vi "MainControl.vi"(9 "Slide":refnum<vi>, 10 "notifier in":refnum<notifier>, 11 "queue in":refnum<queue>) -> ()   [LabVIEW 2013, in "main.lvlib"]
uses:
  main.lvlib
  Controls/Enum User Events.ctl
  <vilib>/DAQmx/write.llb/DAQmx Write (Digital 1D Bool NChan 1Samp 1Line).vi
  <vilib>/DAQmx/create/channels.llb/DAQmx Create Channel (DO-Digital Output).vi
  <vilib>/DAQmx/miscellaneous.llb/DAQmx Fill In Error Info.vi
  Globals/DataAcqRecordPathGlobal.vi
panel:
  in  "Offset":dbl
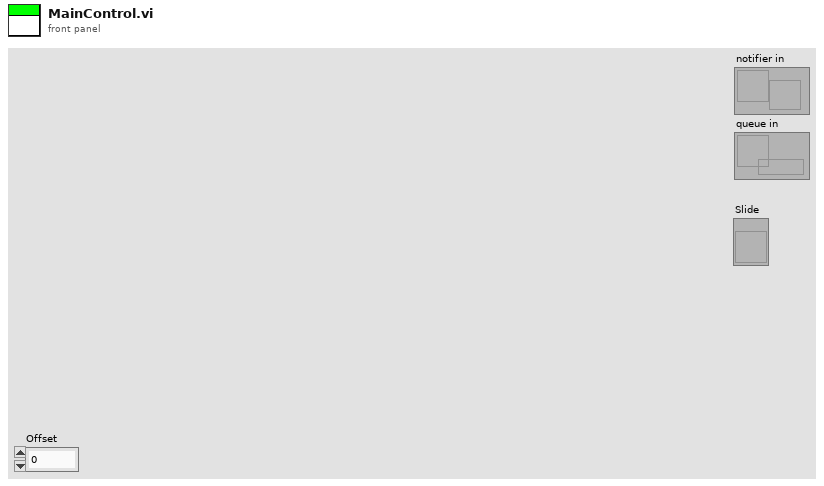
[diagram p1: front panel]
types:
  T1 = typedef "main.lvlib/Enum User Events.ctl" = enum16{"User Event", "Init"}
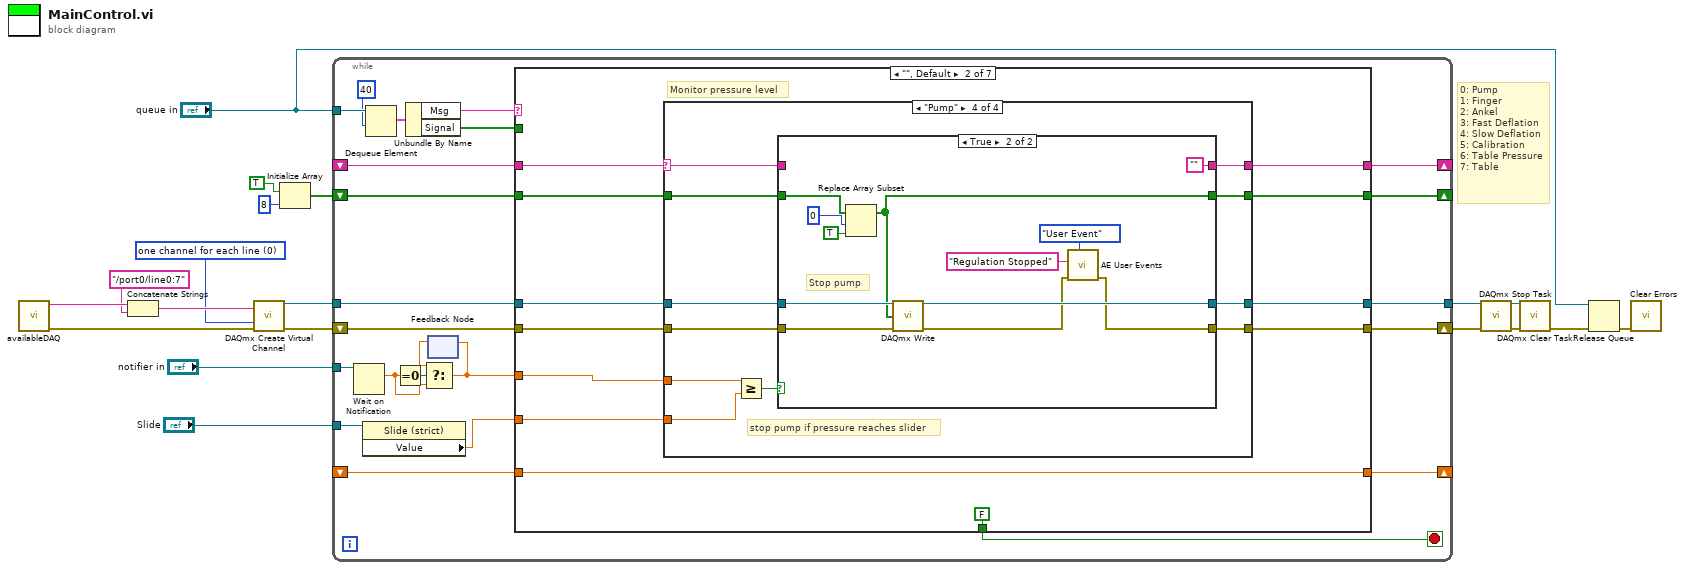
[diagram p0: block diagram]
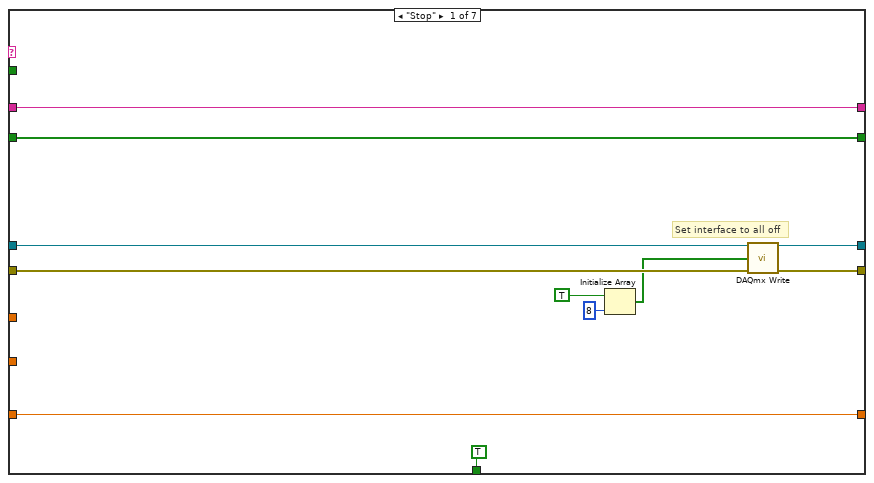
[diagram p2: hidden frame]
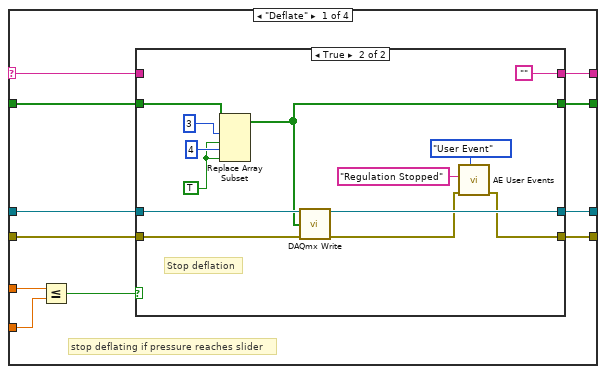
[diagram p3: hidden frame]
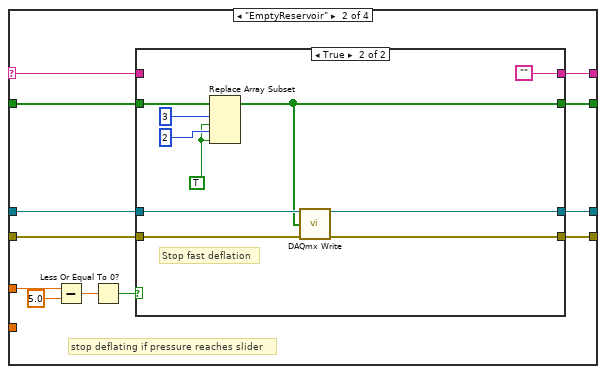
[diagram p5: hidden frame]
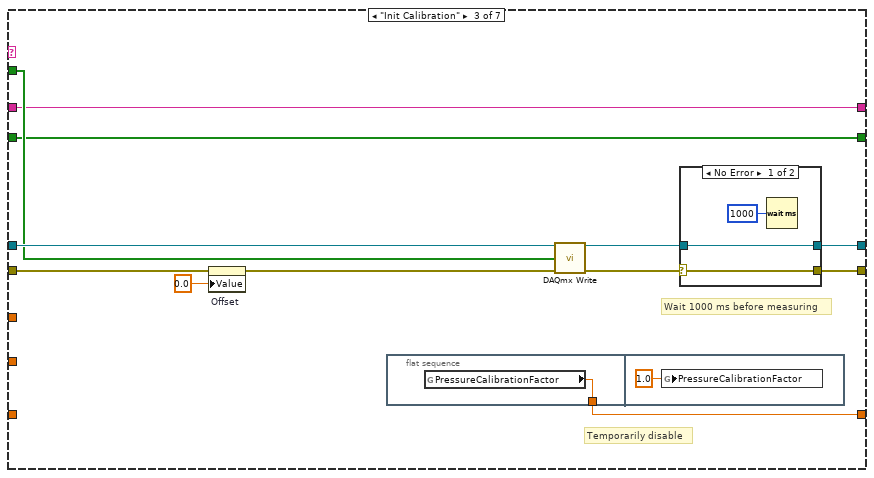
[diagram p9: hidden frame]
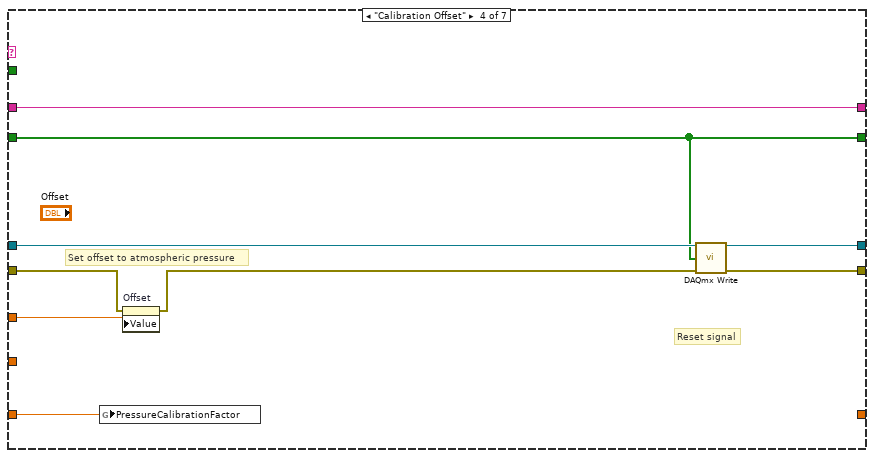
[diagram p11: hidden frame]
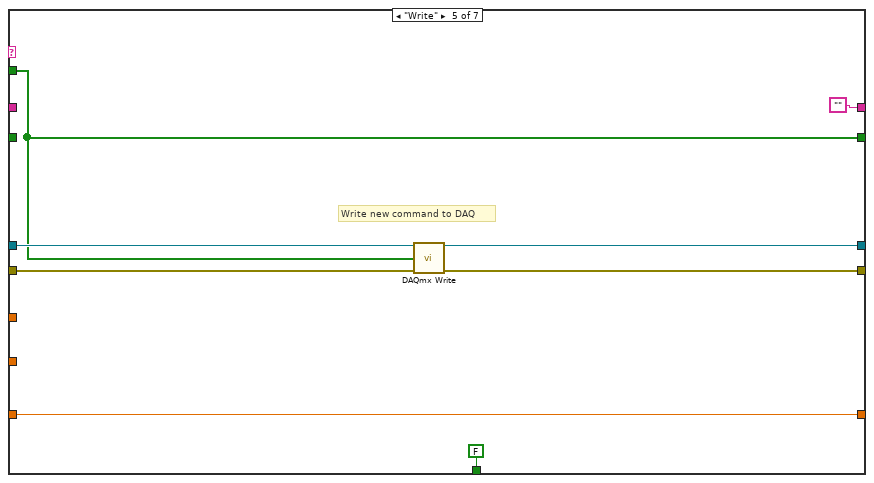
[diagram p12: hidden frame]
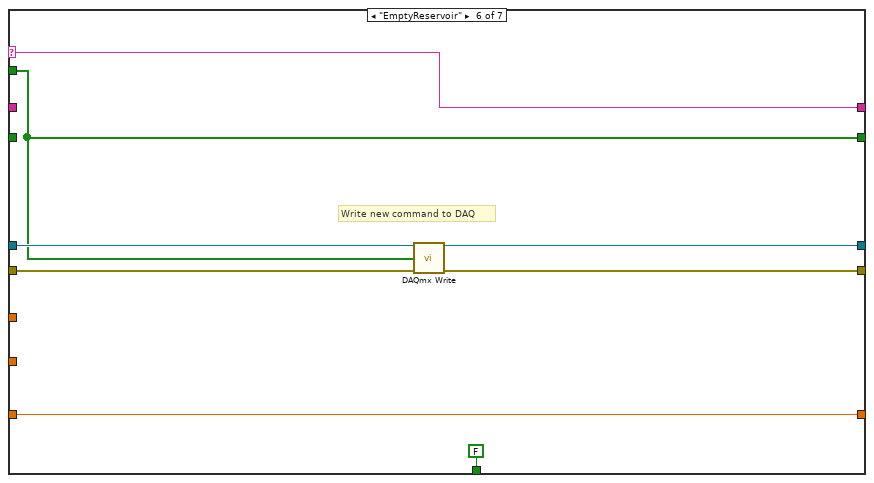
[diagram p13: hidden frame]
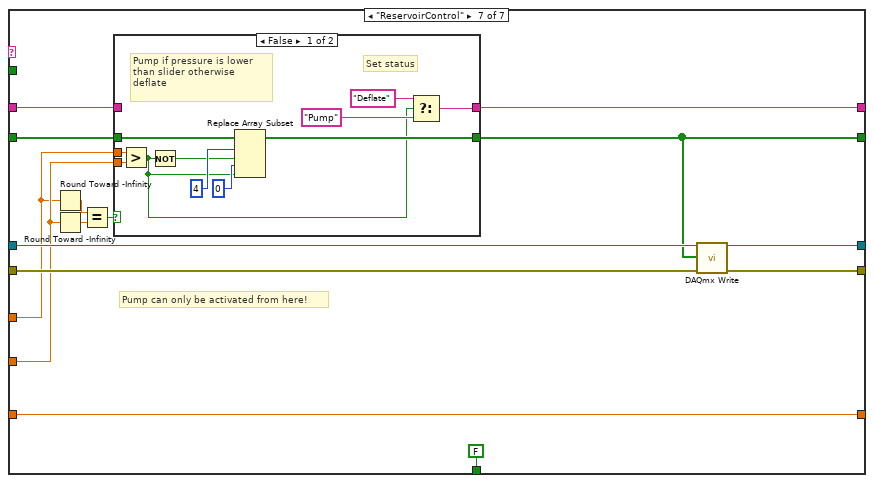
[diagram p14: hidden frame]
diagram:
  w9 = 0 items=["one channel for each line", "one channel for all lines"] ("line grouping")
  # "0: Pump\n1: Finger\n2: Ankel\n3: Fast Deflation\n4: Slow Deflation\n5: Calibration\n6: Table Pressure\n7: Table"
  n1 = call "availableDAQ.vi"() -> ("error out"=w17:errorcluster, "DAQmx Device Name"=w19:tag)  [unwired: 10 in]
  n2 = Concatenate Strings(w19, "/port0/line0:7" ("string")) -> (w16:string)
  n3 = call-poly <vilib>:"DAQmx Create Virtual Channel.vi"("lines"=w16, "line grouping"=w9, "error in"=w17) -> ("task out"=w15:refnum<k21>, "error out"=w14:errorcluster)  [unwired: 11 in]
  n4 = Initialize Array(TRUE, 8 ("dimension size")) -> (w4:bool[])
  n5 = while {
    tunnel: "queue in" -> [w42]
    tunnel: w15 -> [w41]
    shift-right: [w39] -> w12
    shift-left: w14 -> [w40]
    tunnel: [w38] -> w13
    shift-right: [w33] -> _
    shift-left: w4 -> [w32]
    shift-right: [w30] -> _
    shift-left: _ -> [w31]
    shift-right: [w29] -> _
    shift-left: _ -> [w28]
    tunnel: "notifier in" -> [w26]
    tunnel: "Slide" -> [w21]
    stop <- w35 stop-if-true
    n6 = Wait on Notification(notifier=w26) -> (notification=w24:dbl)  [unwired: 3 in, 3 out]
    n7 = property class="Slide (strict)"(reference=w21) -> ("Value"=w20:ext)  [unwired: 1 in, 2 out]
    n8 = Dequeue Element(queue=w42, timeout in ms (-1)=40) -> (element=w37:cluster{"Msg":string, "Signal":bool[]})  [unwired: 1 in, 3 out]
    n9 = Equal To 0?(x=w24) -> (x = 0?=w25:bool)
    n10 = Unbundle By Name(w37) -> ("Msg"=w36:string, "Signal"=w27:bool[])
    n11 = feedback #1() -> (w22:dbl)  [unwired: 1 in]
    n12 = Select(t=w22, s=w25, f=w24) -> (s? t:f=w23:dbl)
    n13 = feedback-in #1(w23) -> ()
    n14 = case shown="\"\", Default" w36 {
      selector: w36 -> [_ _ _ _ _ w188 _]
      tunnel: w41 -> [w49 w64 w162 w175 w186 w194 w209]
      tunnel: w40 -> [w48 w63 w154 w172 w185 w193 w208]
      tunnel: [w50 w61 w157 w176 w183 w191 w206] -> w39
      tunnel: [w51 w62 w155 w177 w184 w192 w207] -> w38
      tunnel: [TRUE FALSE _ _ FALSE FALSE FALSE] -> w35
      tunnel: w27 -> [_ _ w161 _ w181 w189 _]
      tunnel: [w52 w59 w159 w174 w181 w189 w198] -> w33
      tunnel: w32 -> [w52 w60 w159 w174 _ _ w199]
      tunnel: w31 -> [w44 w58 w160 w178 _ _ w196]
      tunnel: w23 -> [_ w57 _ w173 _ _ w200]
      tunnel: w20 -> [_ w56 _ _ _ _ w202]
      tunnel: [w44 w55 w160 w178 "" w188 w197] -> w30
      tunnel: [w43 w54 w151 _ w179 w187 w195] -> w29
      tunnel: w28 -> [w43 w54 _ w170 w179 w187 w195]
      frame "Stop" {
        # "Set interface to all off"
        n15 = Initialize Array(TRUE, 8 ("dimension size")) -> (w45:bool[])
        n16 = call-poly <vilib>:"DAQmx Write.vi"("task/channels in"=w49, "data"=w45, "error in"=w48) -> ("task out"=w51:refnum<k21>, "error out"=w50:errorcluster)  [unwired: 10 in, 1 out]
      }
      frame "", Default {
        # "Monitor pressure level"
        n17 = case shown="\"Pump\"" w58 {
          selector: w58 -> [w67 w98 w123 w125]
          tunnel: w64 -> [w71 w100 w121 w134]
          tunnel: w63 -> [w72 w101 w120 w133]
          tunnel: [w74 w103 w121 w132] -> w62
          tunnel: [w73 w102 w120 w131] -> w61
          tunnel: w60 -> [w76 w105 w122 w129]
          tunnel: [w75 w104 w122 w128] -> w59
          tunnel: [w68 w99 w123 w124] -> w55
          tunnel: w57 -> [w69 w96 _ w127]
          tunnel: w56 -> [w70 _ _ w126]
          frame "Deflate" {
            # "stop deflating if pressure reaches slider"
            n18 = Less Or Equal?(x=w69, y=w70) -> (x <= y?=w66:bool)
            n19 = case shown="True" w66 {
              tunnel: w71 -> [w80 w93]
              tunnel: w72 -> [w79 w92]
              tunnel: [w80 w91] -> w74
              tunnel: [w79 w84] -> w73
              tunnel: w76 -> [w78 w90]
              tunnel: [w78 w81] -> w75
              tunnel: [w77 ""] -> w68
              tunnel: w67 -> [w77 _]
              frame False {
              }
              frame True {
                w82 = TRUE ("new element/subarray")
                # "Stop deflation"
                n20 = Replace Array Subset(array=w90, new element #1=w82, index #1=3 ("index"), new element #2=w82, index #2=4) -> (w81:bool[])
                n21 = call-poly <vilib>:"DAQmx Write.vi"("task/channels in"=w93, "data"=w81, "error in"=w92) -> ("task out"=w91:refnum<k21>, "error out"=w85:errorcluster)  [unwired: 10 in, 1 out]
                n22 = call "AE User Events.vi"("Action"=Enum_User_Events."User Event", "error in (no error)"=w85, "User Event"="Regulation Stopped") -> ("error out"=w84:errorcluster)  [unwired: 7 in, 1 out]
              }
            }
          }
          frame "EmptyReservoir" {
            # "stop deflating if pressure reaches slider"
            n23 = Subtract(x=w96, y=5.0) -> (x-y=w95:dbl)
            n24 = Less Or Equal To 0?(x=w95) -> (x <= 0?=w97:bool)
            n25 = case shown="True" w97 {
              tunnel: w100 -> [w109 w119]
              tunnel: w101 -> [w108 w118]
              tunnel: [w109 w117] -> w103
              tunnel: [w108 w113] -> w102
              tunnel: w105 -> [w107 w116]
              tunnel: [w107 w110] -> w104
              tunnel: [w106 ""] -> w99
              tunnel: w98 -> [w106 _]
              frame False {
              }
              frame True {
                w111 = TRUE ("new element/subarray")
                # "Stop fast deflation"
                n26 = Replace Array Subset(array=w116, new element #1=w111, index #1=3 ("index"), new element #2=w111, index #2=2 ("index")) -> (w110:bool[])
                n27 = call-poly <vilib>:"DAQmx Write.vi"("task/channels in"=w119, "data"=w110, "error in"=w118) -> ("task out"=w117:refnum<k21>, "error out"=w113:errorcluster)  [unwired: 10 in, 1 out]
              }
            }
          }
          frame "", Default {
          }
          frame "Pump" {
            # "stop pump if pressure reaches slider"
            n28 = Greater Or Equal?(x=w127, y=w126) -> (x >= y?=w130:bool)
            n29 = case shown="True" w130 {
              tunnel: w134 -> [w138 w150]
              tunnel: w133 -> [w137 w149]
              tunnel: [w138 w148] -> w132
              tunnel: [w137 w142] -> w131
              tunnel: w129 -> [w136 w145]
              tunnel: [w136 w139] -> w128
              tunnel: w125 -> [w135 _]
              tunnel: [w135 ""] -> w124
              frame False {
              }
              frame True {
                # "Stop pump"
                n30 = Replace Array Subset(array=w145, new element=TRUE ("new element/subarray"), index=0) -> (w139:bool[])
                n31 = call-poly <vilib>:"DAQmx Write.vi"("task/channels in"=w150, "data"=w139, "error in"=w149) -> ("task out"=w148:refnum<k21>, "error out"=w143:errorcluster)  [unwired: 10 in, 1 out]
                n32 = call "AE User Events.vi"("Action"=Enum_User_Events."User Event", "error in (no error)"=w143, "User Event"="Regulation Stopped") -> ("error out"=w142:errorcluster)  [unwired: 7 in, 1 out]
              }
            }
          }
        }
      }
      frame "Init Calibration" {
        # "Temporarily disable"
        # "Wait 1000 ms before measuring"
        n33 = property on="Offset" class="DigNum (strict)"(error in=w154, "Value"=0.0 ("Offset")) -> (error out=w153:errorcluster)  [unwired: 1 in, 1 out]
        n34 = flat-sequence {
          tunnel: [w163] -> w151
          frame #0 {
            n35 = global read "DataAcqRecordPathGlobal.vi" "PressureCalibrationFactor"() -> (w163:dbl)
          }
          frame #1 {
            n36 = global write "DataAcqRecordPathGlobal.vi" "PressureCalibrationFactor"(1.0 ("PressureCalibrationFactor")) -> ()
          }
        }
        n37 = call-poly <vilib>:"DAQmx Write.vi"("task/channels in"=w162, "data"=w161, "error in"=w153) -> ("task out"=w156:refnum<k21>, "error out"=w158:errorcluster)  [unwired: 10 in, 1 out]
        n38 = case shown="No Error" w158 {
          selector: w158 -> [w167 w169]
          tunnel: [w167 w169] -> w157
          tunnel: [w166 w168] -> w155
          tunnel: w156 -> [w166 w168]
          frame No Error {
            n39 = Wait (ms)(milliseconds to wait=u32 1000) -> ()  [unwired: 1 out]
          }
          frame Error {
          }
        }
      }
      frame "Calibration Offset" {
        # "Reset signal"
        # "Set offset to atmospheric pressure"
        n40 = global write "DataAcqRecordPathGlobal.vi" "PressureCalibrationFactor"(w170) -> ()
        n41 = property on="Offset" class="DigNum (strict)"(error in=w172, "Value"=w173) -> (error out=w171:errorcluster)  [unwired: 1 in, 1 out]
        n42 = call-poly <vilib>:"DAQmx Write.vi"("task/channels in"=w175, "data"=w174, "error in"=w171) -> ("task out"=w177:refnum<k21>, "error out"=w176:errorcluster)  [unwired: 10 in, 1 out]
      }
      frame "Write" {
        # "Write new command to DAQ"
        n43 = call-poly <vilib>:"DAQmx Write.vi"("task/channels in"=w186, "data"=w181, "error in"=w185) -> ("task out"=w184:refnum<k21>, "error out"=w183:errorcluster)  [unwired: 10 in, 1 out]
      }
      frame "EmptyReservoir" {
        # "Write new command to DAQ"
        n44 = call-poly <vilib>:"DAQmx Write.vi"("task/channels in"=w194, "data"=w189, "error in"=w193) -> ("task out"=w192:refnum<k21>, "error out"=w191:errorcluster)  [unwired: 10 in, 1 out]
      }
      frame "ReservoirControl" {
        # "Pump can only be activated from here!"
        n45 = Round Toward -Infinity(1:w200) -> (0:w201:dbl)
        n46 = Round Toward -Infinity(1:w202) -> (0:w203:ext)
        n47 = Equal?(x=w201, y=w203) -> (x = y?=w204:bool)
        n48 = case shown="False" w204 {
          tunnel: w199 -> [w220 w222]
          tunnel: w200 -> [w218 _]
          tunnel: w202 -> [w217 _]
          tunnel: [w213 w222] -> w198
          tunnel: [w214 w221] -> w197
          tunnel: w196 -> [_ w221]
          frame False {
            # "Set status"
            # "Pump if pressure is lower than slider otherwise deflate"
            n49 = Greater?(x=w218, y=w217) -> (0:w211:bool)
            n50 = Not(x=w211) -> (.not. x?=w215:bool)
            n51 = Replace Array Subset(array=w220, new element #1=w215, index #1=4 ("index"), new element #2=w211, index #2=0 ("index")) -> (w213:bool[])
            n52 = Select(t="Deflate", s=w211, f="Pump") -> (s? t:f=w214:string)
          }
          frame True {
            # "Ignore if pressure = slide"
          }
        }
        n53 = call-poly <vilib>:"DAQmx Write.vi"("task/channels in"=w209, "data"=w198, "error in"=w208) -> ("task out"=w207:refnum<k21>, "error out"=w206:errorcluster)  [unwired: 10 in, 1 out]
      }
    }
  }
  n54 = call <vilib>:"DAQmx Stop Task.vi"("task/channels in"=w13, "error in"=w12) -> ("task out"=w11:refnum<k21>, "error out"=w10:errorcluster)  [unwired: 12 in]
  n55 = call <vilib>:"DAQmx Clear Task.vi"("task in"=w11, "error in"=w10) -> ("error out"=w8:errorcluster)  [unwired: 13 in]
  n56 = Release Queue(queue="queue in", error in (no error)=w8) -> (error out=w7:errorcluster)  [unwired: 1 in, 2 out]
  n57 = call <vilib>:"Clear Errors.vi"("error in (no error)"=w7) -> ()  [unwired: 6 in, 1 out]
